vi "Set Sub Objects Dictionary.vi"(8 "error in (no error)":errorcluster, 10 "Sub Objects Dictionary":refnum<class "Sub Objects Dictionary.lvclass">, 11 "Object Entry in":refnum<class "Object Entry.lvclass">) -> (0 "error out":errorcluster, 3 "Object Entry out":refnum<class "Object Entry.lvclass">)   [LabVIEW 2020, in "CANopen.lvlib" / "Object Entry.lvclass"]
uses:
  Object Entry.lvclass
  Sub Objects Dictionary/Sub Objects Dictionary.lvclass
  Object Entry.lvclass/Object Entry.ctl
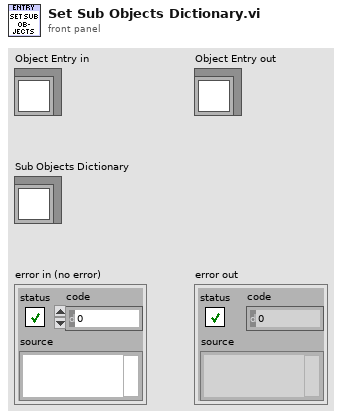
[diagram p1: front panel]
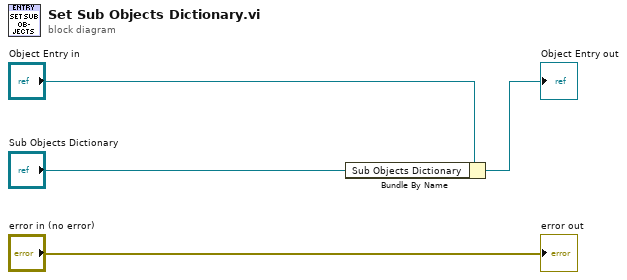
[diagram p0: block diagram]
diagram:
  n1 = Bundle By Name(cluster="Object Entry in", "Sub Objects Dictionary"="Sub Objects Dictionary") -> (→"Object Entry out":refnum<class "Object Entry.lvclass">)
  "error out" <- "error in (no error)"
